vi "main.vi"() -> ()   [LabVIEW 2017]
panel:
  in  "stop get state":bool
  out "Robot mode":T1(ring)
  out "client out byte array":u8[](array[numeric])
  out "state client out":string
  out "state error out 2":errorcluster
  out "Robot mode":T1(ring)
  out "speed cmd string":string
  out "JointMovJ string":string
  in  "j4-":bool
  in  "j3-":bool
  in  "j2-":bool
  in  "j1-":bool
  in  "j4+":bool
  in  "j3+":bool
  in  "j2+":bool
  in  "j1+":bool
  out "client out byte array":u8[](array[numeric])
  out "state error out":errorcluster
  out "state client out":string
  in  "Robot State":bool
  out "error out":errorcluster
  in  "Start trace":bool
  in  "tracePath":string
  in  "Stop move":bool
  in  "JointMovJ":bool
  in  "j4":dbl
  in  "j3":dbl=100.0
  in  "j2":dbl
  in  "j1":dbl
  in  "Speed confrim":bool
  in  "Speed Factor":dbl
  in  "Emergency Stop":bool
  in  "Power up":bool
  out "data out":string
  in  "ClearError":bool
  in  "Enable button":bool
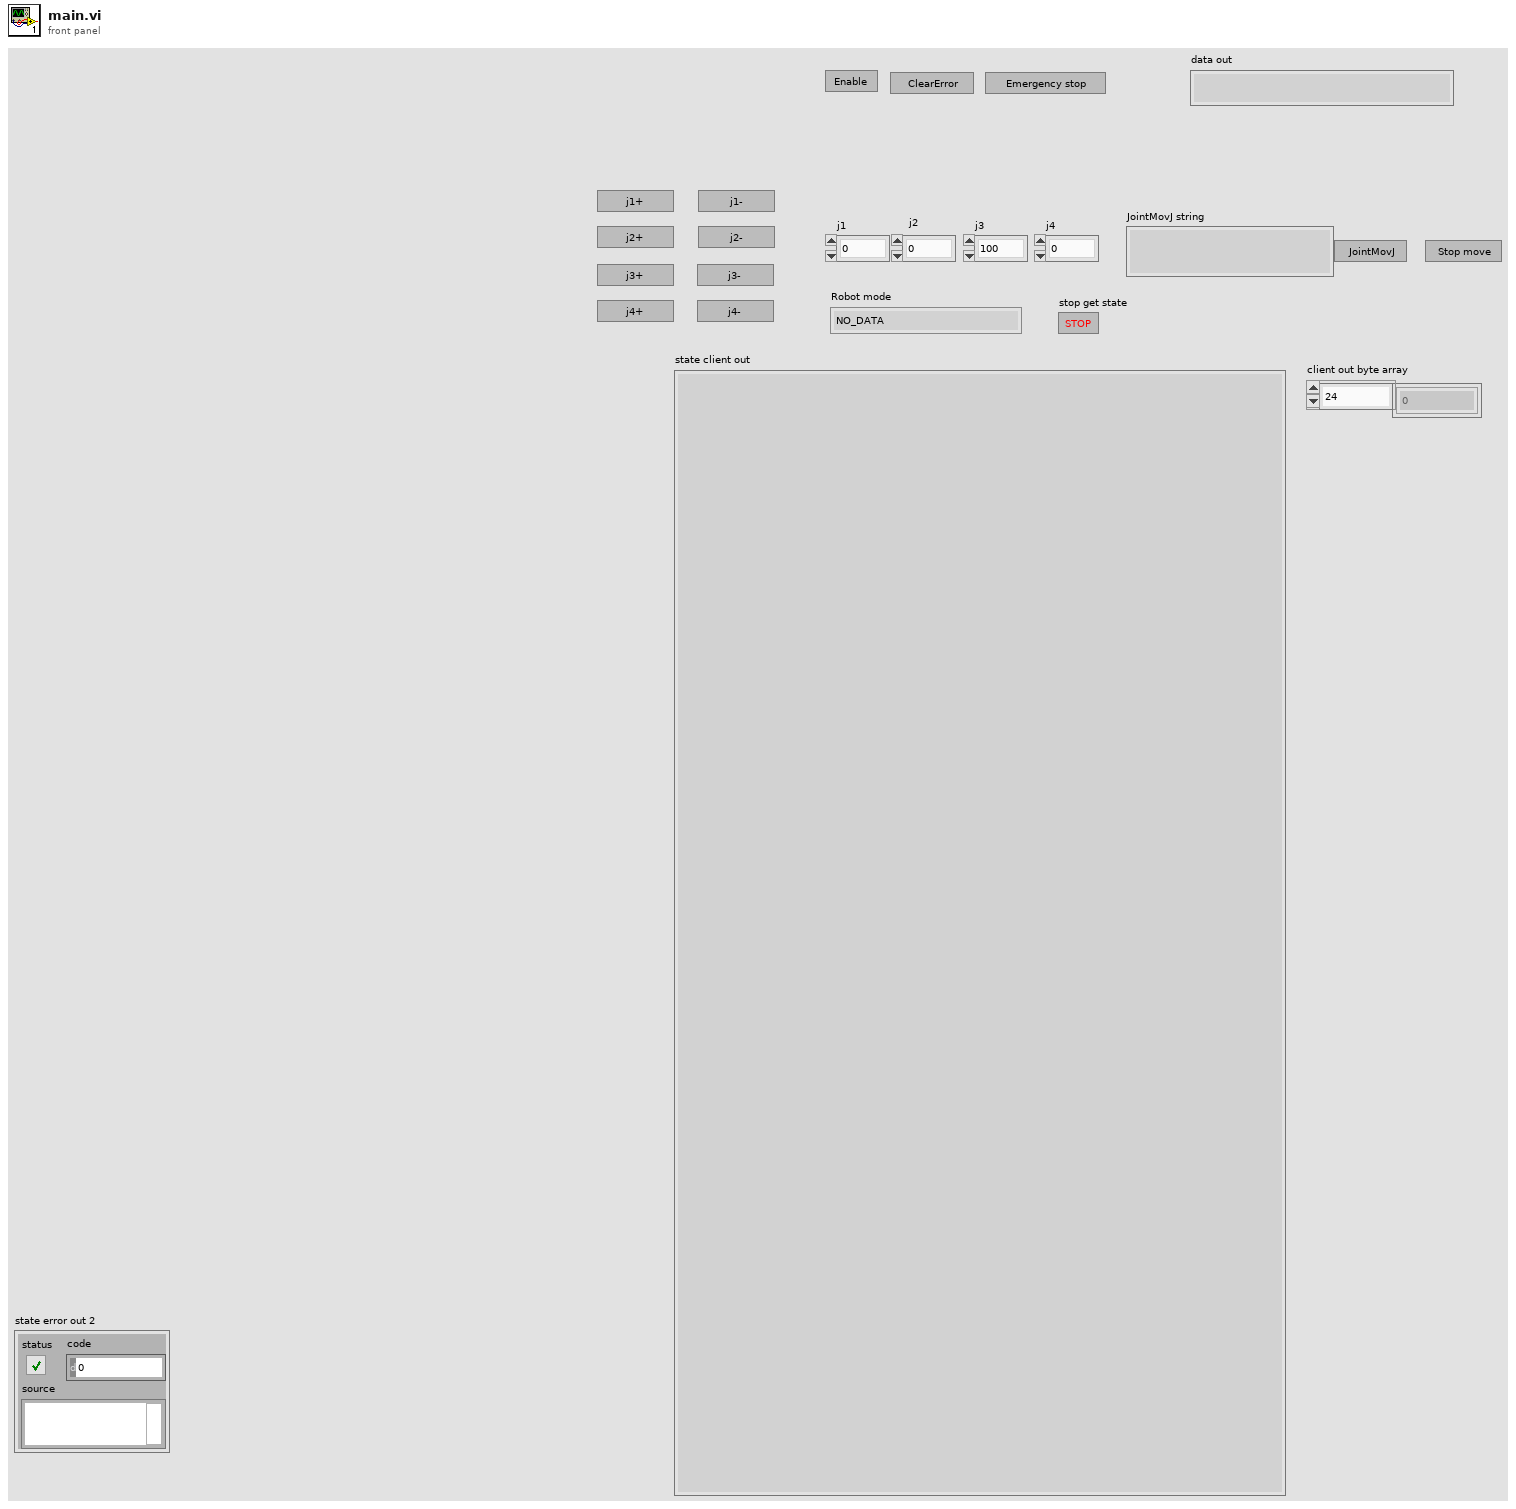
[diagram p1: front panel]
types:
  T1 = enum16{"NO_DATA", "ROBOT_MODE_INIT", "ROBOT_MODE_BRAKE_OPEN", "HOLD_BITS", "ROBOT_MODE_DISABLED", "ROBOT_MODE_ENABLE", "ROBOT_MODE_BACKDRIVE", "ROBOT_MODE_RUNNING", "ROBOT_MODE_RECORDING", "ROBOT_MODE_ERROR", "ROBOT_MODE_PAUSE", "ROBOT_MODE_JOG"}
  T2 = enum16{"Standard", "Buffered", "CRLF", "Immediate"}
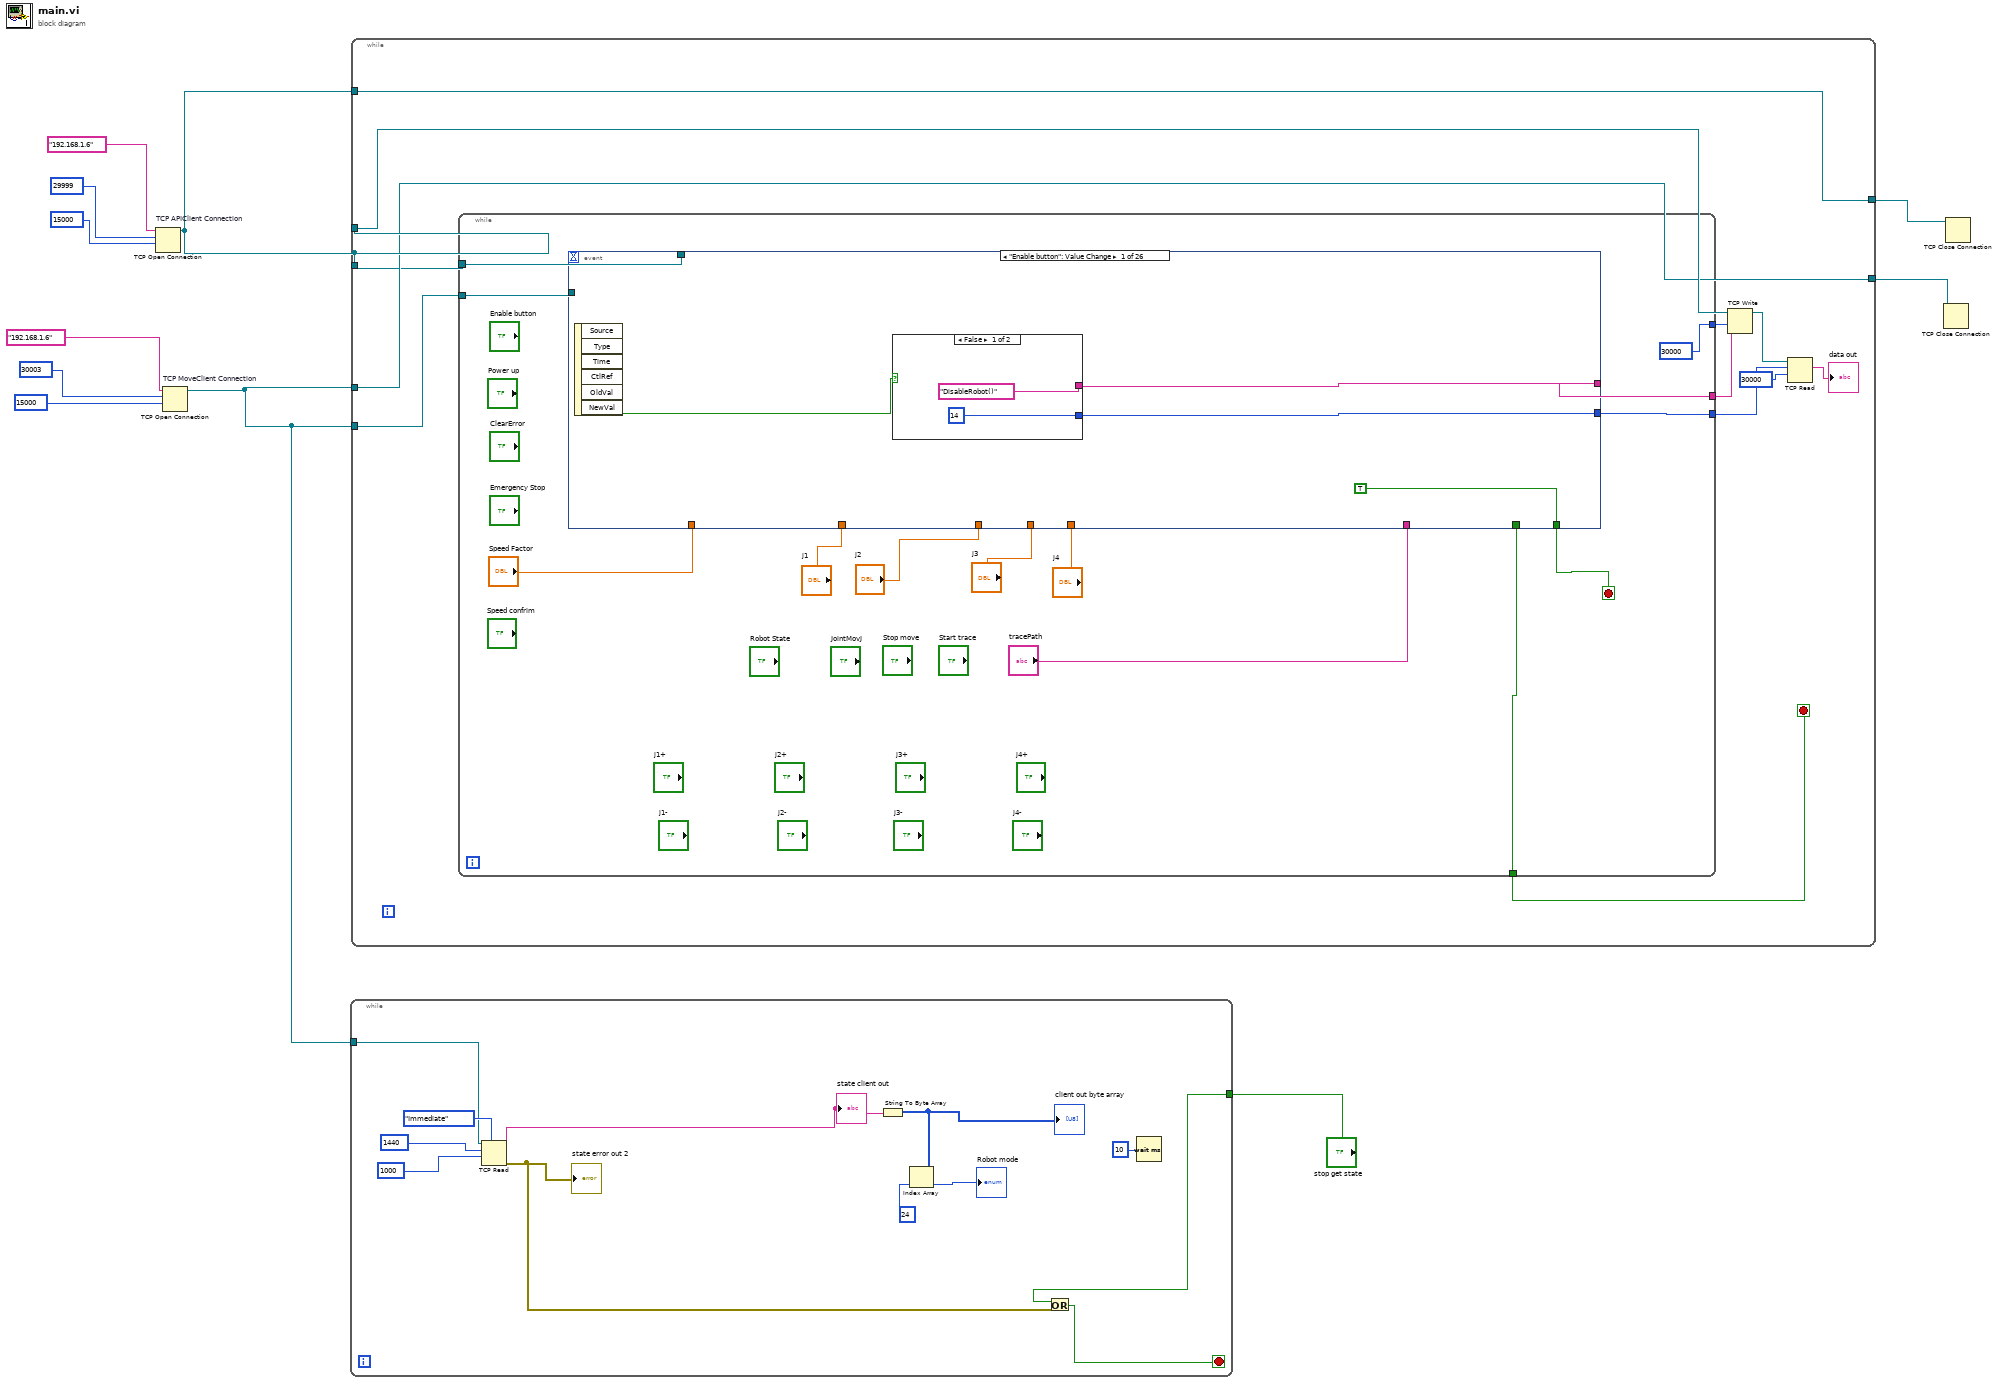
[diagram p0: block diagram]
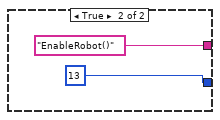
[diagram p2: hidden frame]
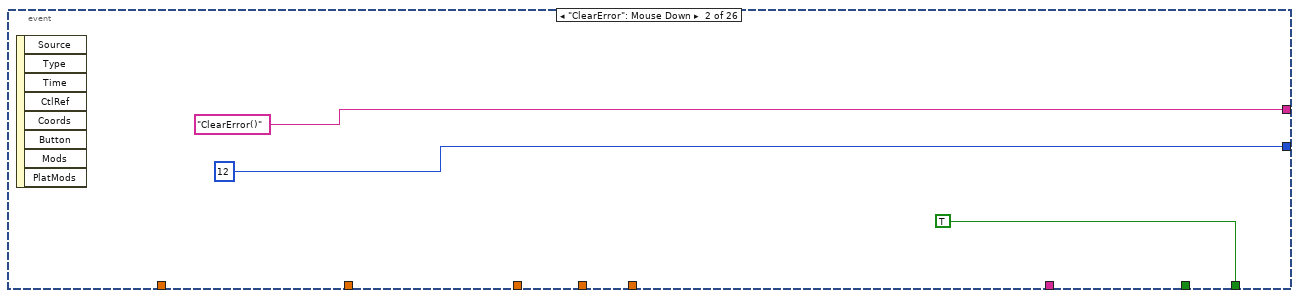
[diagram p3: hidden frame]
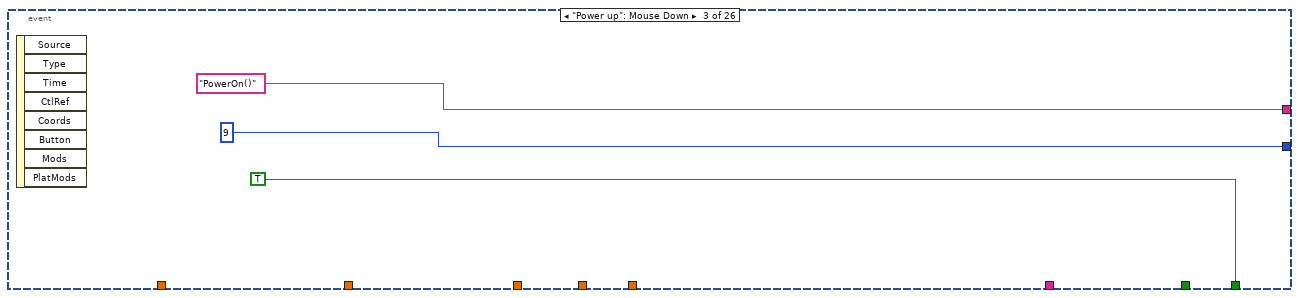
[diagram p4: hidden frame]
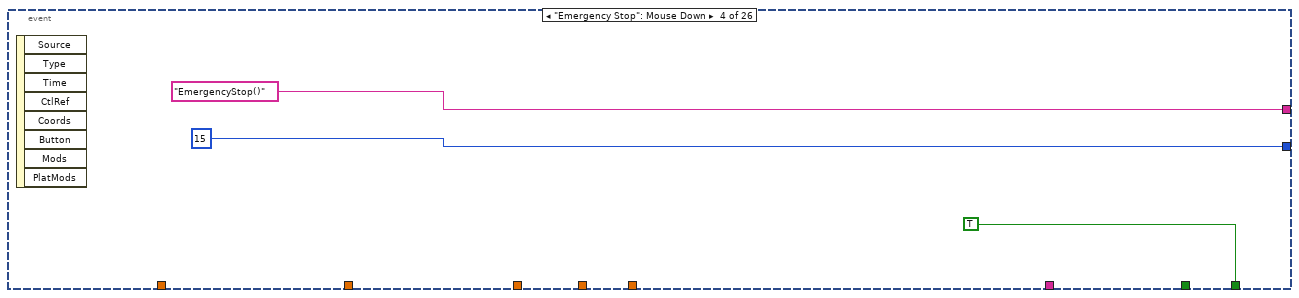
[diagram p5: hidden frame]
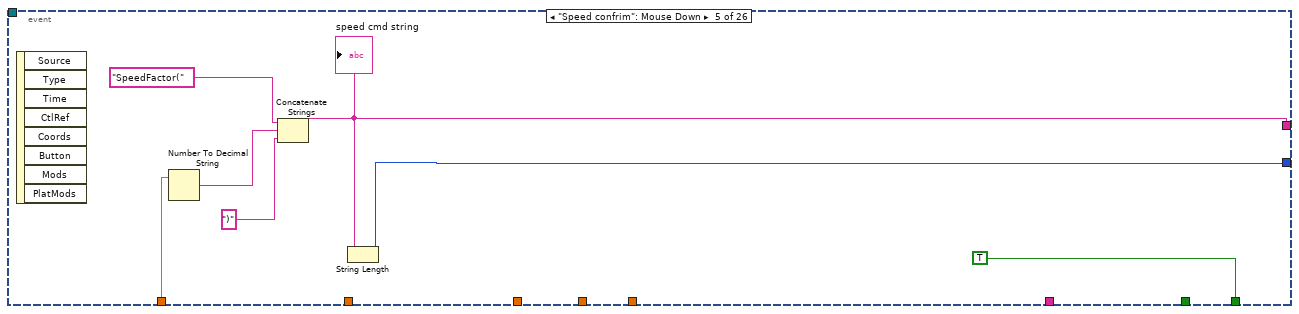
[diagram p6: hidden frame]
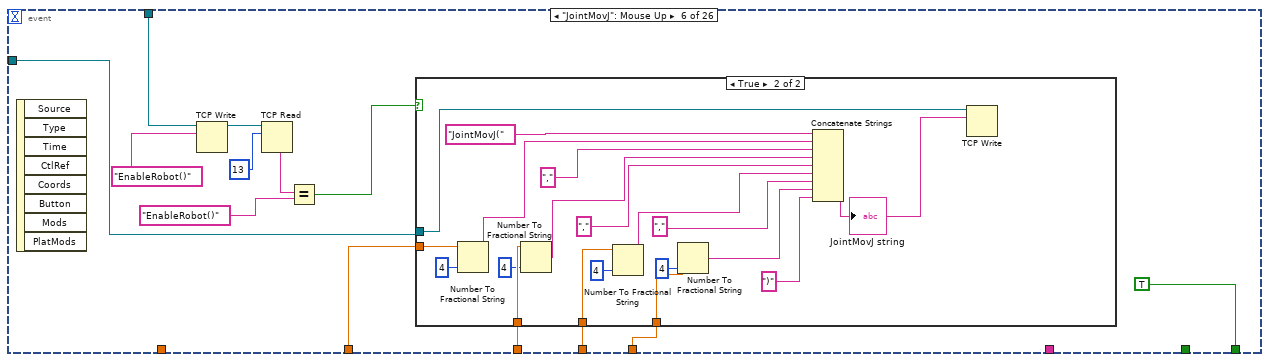
[diagram p7: hidden frame]
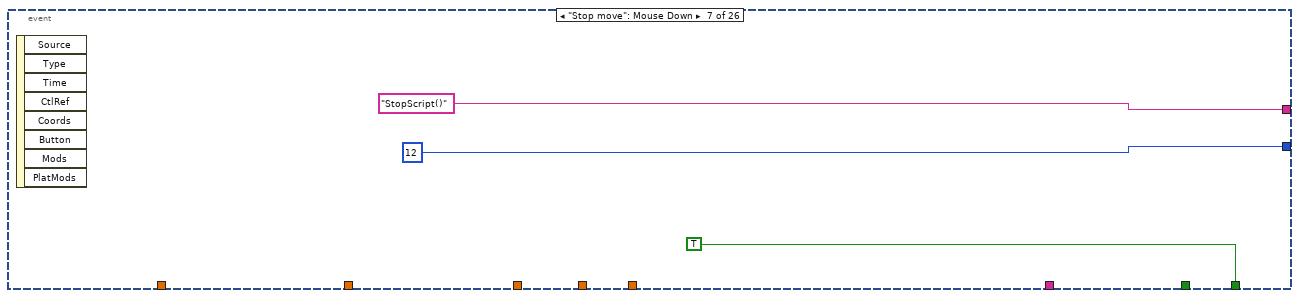
[diagram p9: hidden frame]
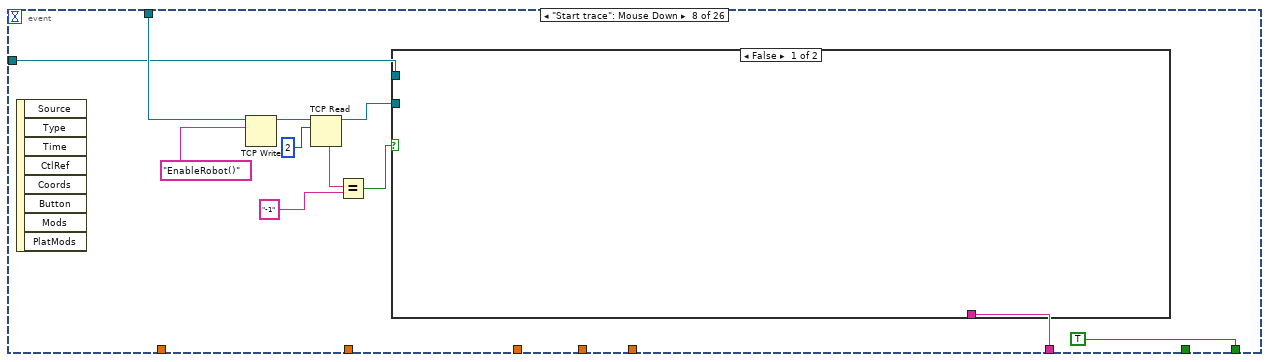
[diagram p10: hidden frame]
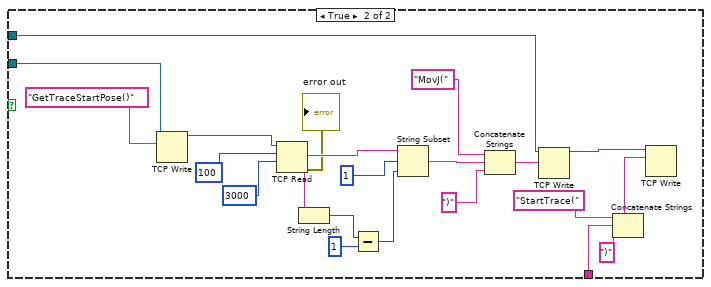
[diagram p11: hidden frame]
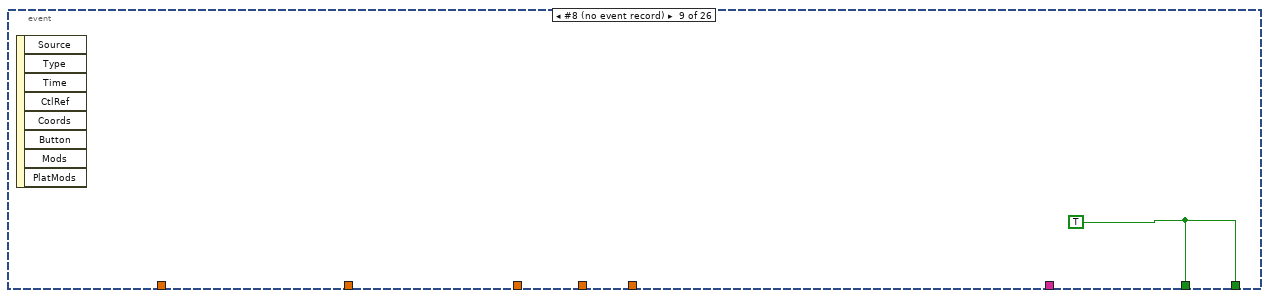
[diagram p12: hidden frame]
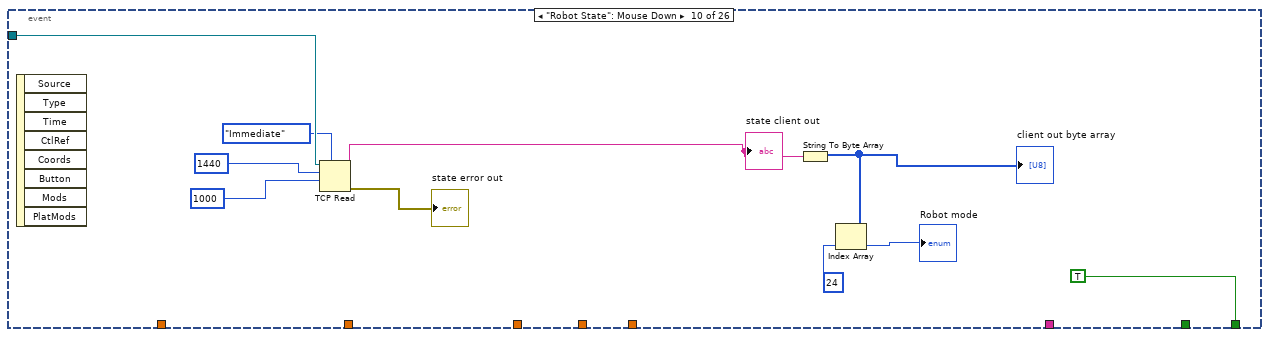
[diagram p13: hidden frame]
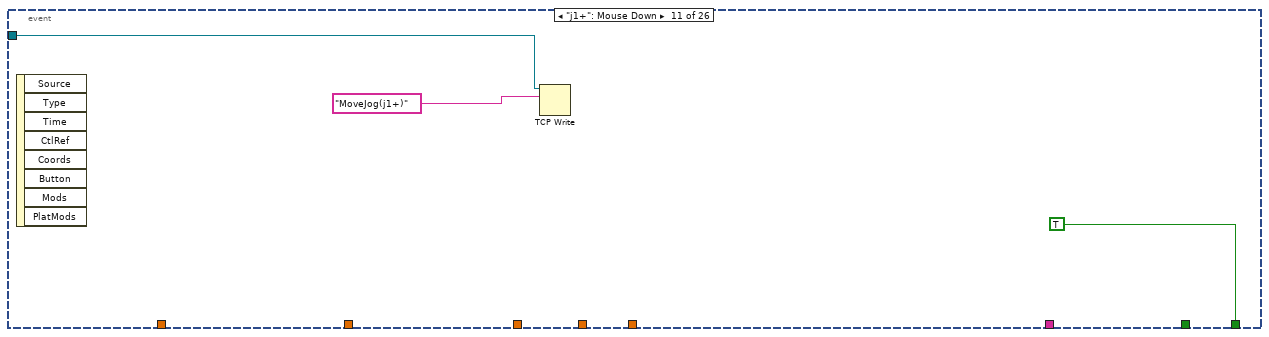
[diagram p14: hidden frame]
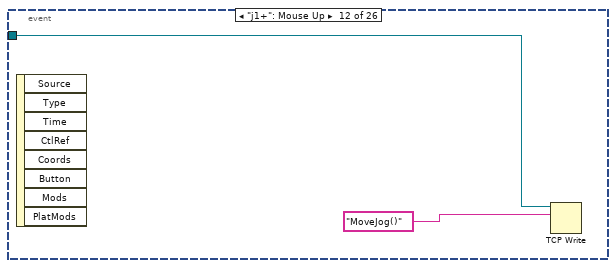
[diagram p15: hidden frame]
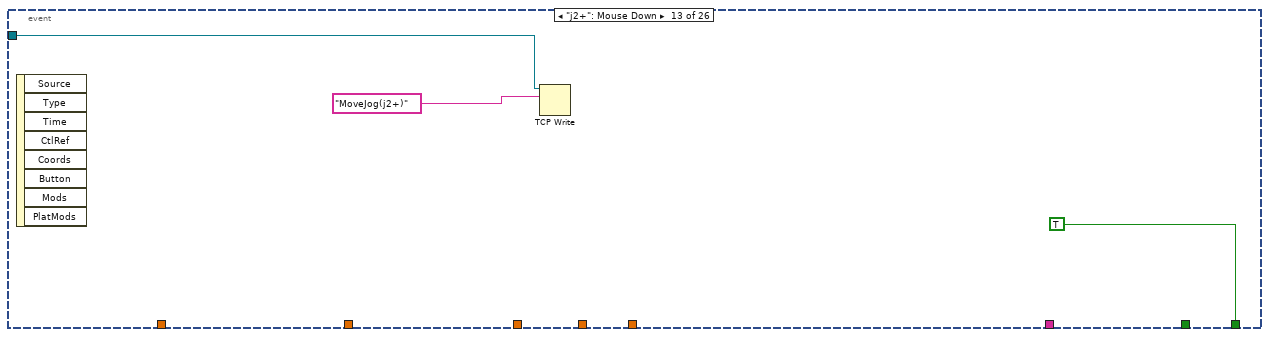
[diagram p16: hidden frame]
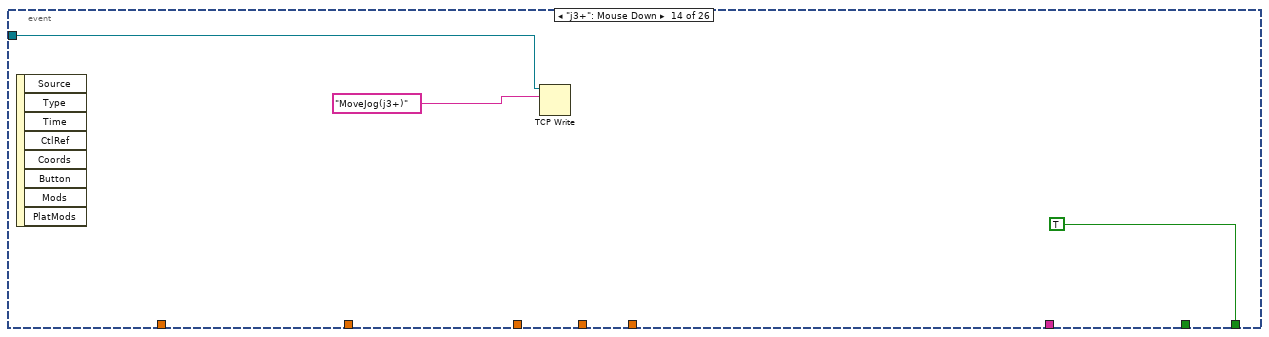
[diagram p17: hidden frame]
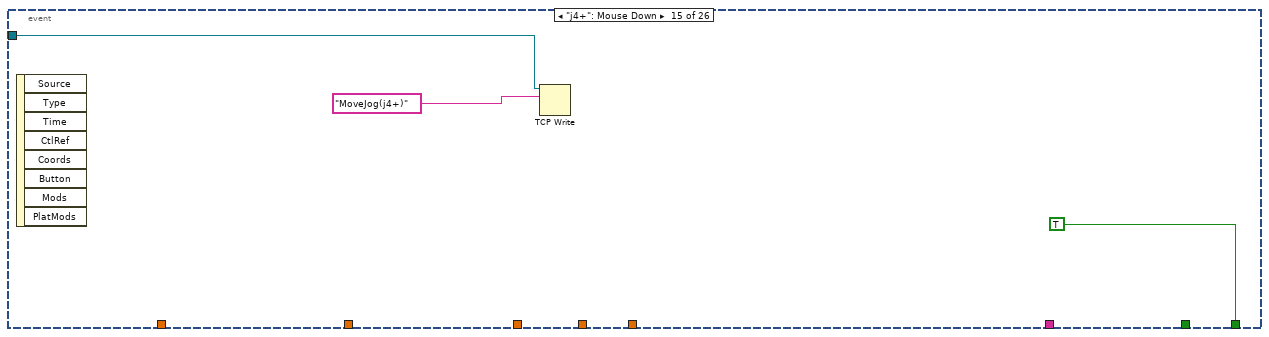
[diagram p18: hidden frame]
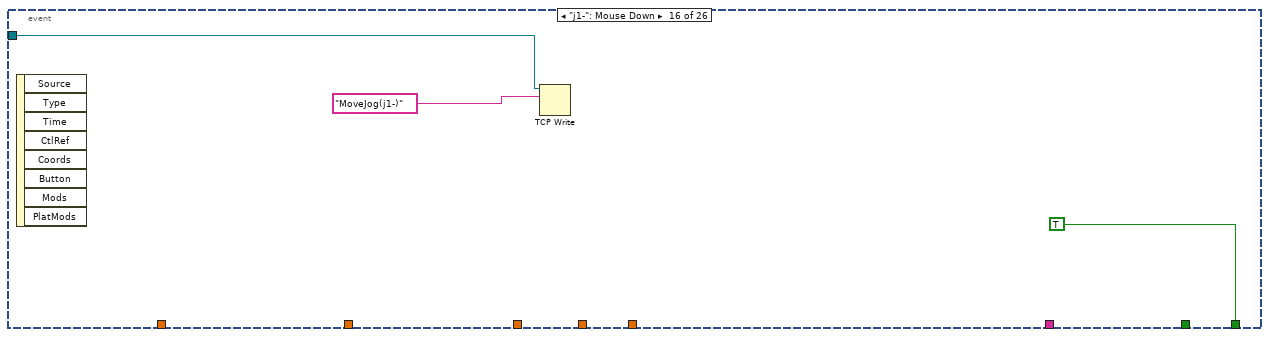
[diagram p19: hidden frame]
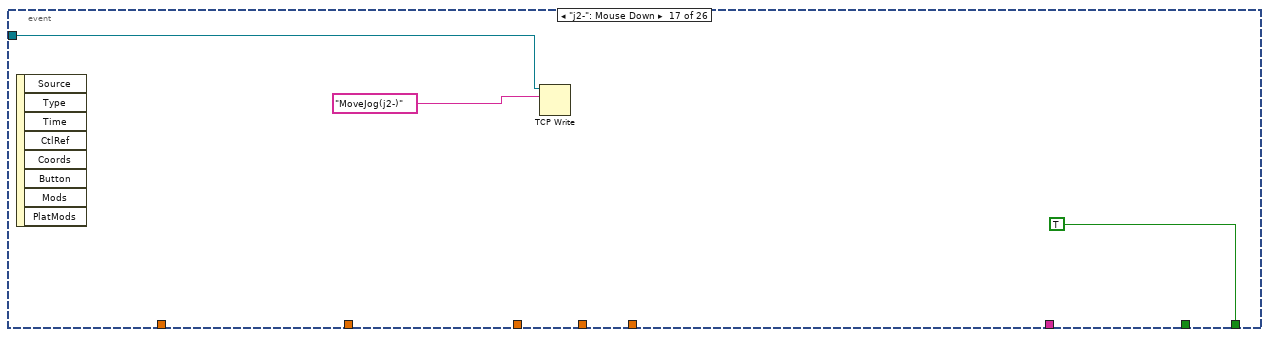
[diagram p20: hidden frame]
diagram:
  n1 = TCP Open Connection "TCP APIClient Connection"(address="192.168.1.6", remote port or service name=29999, timeout ms (60000)=15000) -> (connection ID=w3:refnum<k5>)  [unwired: 2 in, 1 out]
  n2 = TCP Open Connection "TCP MoveClient Connection"(address="192.168.1.6", remote port or service name=30003, timeout ms (60000)=15000) -> (connection ID=w2:refnum<k5>)  [unwired: 2 in, 1 out]
  n3 = while {
    tunnel: w2 -> [w20]
    tunnel: "stop get state" -> [w14]
    stop <- w13 stop-if-true
    n4 = TCP Read(connection ID=w20, bytes to read=1440, 7:T2."Immediate" ("mode (standard)"), 9:1000 ("timeout ms (25000)")) -> (data out=w16:string, error out=w12:errorcluster)  [unwired: 1 in, 1 out]
    "state error out 2" <- w12
    "state client out" <- w16
    n5 = String To Byte Array(string=w16) -> (unsigned byte array=w19:u8[])
    "client out byte array" <- w19
    n6 = Index Array(array=w19, index=24) -> (element=→"Robot mode":u8)
    n7 = Or(x=w14, y=w12) -> (x .or. y?=w13:bool)
    n8 = Wait (ms)(milliseconds to wait=u32 10) -> ()  [unwired: 1 out]
  }
  n9 = while {
    tunnel: w3 -> [w34]
    tunnel: [w30] -> w5
    tunnel: w2 -> [w30]
    tunnel: [w29] -> w4
    tunnel: w3 -> [w29]
    tunnel: w3 -> [w28]
    tunnel: w2 -> [w27]
    stop <- w26 stop-if-true
    n10 = while {
      tunnel: [w41] -> w35
      tunnel: [w48] -> w32
      tunnel: w28 -> [w46]
      tunnel: w27 -> [w45]
      tunnel: [w38] -> w26
      tunnel: [30000 ("timeout ms (25000)")] -> w24
      stop <- w39 stop-if-true
      n11 = event shown="[0] \"Enable button\": Value Change" {
        selector: _ -> [_ _ _ _ _ _ _ _ _ _ _ _ _ _ _ _ _ _ _ _ _ _ _ _ _ _]
        dyn-events: _ -> [_ _ _ _ _ _ _ _ _ _ _ _ _ _ _ _ _ _ _ _ _ _ _ _ _ _]
        timeout: _ -> [_ _ _ _ _ _ _ _ _ _ _ _ _ _ _ _ _ _ _ _ _ _ _ _ _ _]
        tunnel: [w52 "ClearError()" "PowerOn()" "EmergencyStop()" w68 _ "StopScript()" _ _ _ _ _ _ _ _ _ _ _ _ _ _ _ _ _ _ _] -> w41
        tunnel: [w51 12 9 15 w70 _ 12 _ _ _ _ _ _ _ _ _ _ _ _ _ _ _ _ _ _ _] -> w48
        tunnel: "Speed Factor" -> [_ _ _ _ w72 _ _ _ _ _ _ _ _ _ _ _ _ _ _ _ _ _ _ _ _ _]
        tunnel: w46 -> [_ _ _ _ _ w85 _ w113 _ _ _ _ _ _ _ _ _ _ _ _ _ _ _ _ _ _]
        tunnel: w45 -> [_ _ _ _ _ w79 _ w110 _ w146 w151 w154 w156 w159 w162 w165 w168 w171 w174 w177 w179 w181 w183 w185 w187 w189]
        tunnel: "j1" -> [_ _ _ _ _ w78 _ _ _ _ _ _ _ _ _ _ _ _ _ _ _ _ _ _ _ _]
        tunnel: "j2" -> [_ _ _ _ _ w77 _ _ _ _ _ _ _ _ _ _ _ _ _ _ _ _ _ _ _ _]
        tunnel: "j3" -> [_ _ _ _ _ w76 _ _ _ _ _ _ _ _ _ _ _ _ _ _ _ _ _ _ _ _]
        tunnel: "j4" -> [_ _ _ _ _ w75 _ _ _ _ _ _ _ _ _ _ _ _ _ _ _ _ _ _ _ _]
        tunnel: "tracePath" -> [_ _ _ _ _ _ _ w109 _ _ _ _ _ _ _ _ _ _ _ _ _ _ _ _ _ _]
        tunnel: [TRUE TRUE TRUE TRUE TRUE TRUE TRUE TRUE w140 TRUE TRUE _ TRUE TRUE TRUE TRUE TRUE TRUE TRUE _ _ _ _ _ _ _] -> w39
        tunnel: [_ _ _ _ _ _ _ _ w140 _ _ _ _ _ _ _ _ _ _ _ _ _ _ _ _ _] -> w38
        event "Enable button": Value Change {
          n12 = event-data() -> ("NewVal"=w49:bool)  [unwired: 1 in, 5 out]
          n13 = case shown="False" w49 {
            tunnel: ["DisableRobot()" "EnableRobot()"] -> w52
            tunnel: [14 13] -> w51
            frame False {
            }
            frame True {
            }
          }
        }
        event "ClearError": Mouse Down {
          n14 = event-data() -> ()  [unwired: 1 in, 8 out]
        }
        event "Power up": Mouse Down {
          n15 = event-data() -> ()  [unwired: 1 in, 8 out]
        }
        event "Emergency Stop": Mouse Down {
          n16 = event-data() -> ()  [unwired: 1 in, 8 out]
        }
        event "Speed confrim": Mouse Down {
          n17 = event-data() -> ()  [unwired: 1 in, 8 out]
          n18 = Number To Decimal String(number=w72) -> (decimal integer string=w67:string)  [unwired: 1 in]
          n19 = Concatenate Strings("SpeedFactor(", w67, ")") -> (w68:string)
          "speed cmd string" <- w68
          n20 = String Length(string=w68) -> (length=w70:i32)
        }
        event "JointMovJ": Mouse Up {
          n21 = event-data() -> ()  [unwired: 1 in, 8 out]
          n22 = TCP Write(connection ID=w85, data in="EnableRobot()") -> (connection ID out=w84:refnum<k5>)  [unwired: 2 in, 2 out]
          n23 = TCP Read(connection ID=w84, bytes to read=13) -> (data out=w81:string)  [unwired: 3 in, 2 out]
          n24 = Equal?(x=w81, y="EnableRobot()") -> (x = y?=w74:bool)
          n25 = case shown="True" w74 {
            tunnel: w79 -> [_ w104]
            tunnel: w78 -> [_ w103]
            tunnel: w77 -> [_ w102]
            tunnel: w76 -> [_ w101]
            tunnel: w75 -> [_ w100]
            frame False {
            }
            frame True {
              n26 = Number To Fractional String(number=w103, precision (6)=i16 4) -> (F-format string=w99:string)  [unwired: 2 in]
              n27 = Number To Fractional String(number=w102, precision (6)=i16 4) -> (F-format string=w95:string)  [unwired: 2 in]
              n28 = Number To Fractional String(number=w101, precision (6)=i16 4) -> (F-format string=w91:string)  [unwired: 2 in]
              n29 = Number To Fractional String(number=w100, precision (6)=i16 4) -> (F-format string=w93:string)  [unwired: 2 in]
              n30 = Concatenate Strings("JointMovJ(" ("string"), w99, "," ("string"), w95, "," ("string"), w91, "," ("string"), w93, ")" ("string")) -> (w86:string)
              "JointMovJ string" <- w86
              n31 = TCP Write(connection ID=w104, data in=w86) -> ()  [unwired: 2 in, 3 out]
            }
          }
        }
        event "Stop move": Mouse Down {
          n32 = event-data() -> ()  [unwired: 1 in, 8 out]
        }
        event "Start trace": Mouse Down {
          n33 = event-data() -> ()  [unwired: 1 in, 8 out]
          n34 = TCP Write(connection ID=w113, data in="EnableRobot()") -> (connection ID out=w118:refnum<k5>)  [unwired: 2 in, 2 out]
          n35 = TCP Read(connection ID=w118, bytes to read=2) -> (connection ID out=w111:refnum<k5>, data out=w115:string)  [unwired: 3 in, 1 out]
          n36 = Equal?(x=w115, y="-1") -> (x = y?=w112:bool)
          n37 = case shown="False" w112 {
            tunnel: w111 -> [_ w138]
            tunnel: w110 -> [_ w125]
            tunnel: w109 -> [_ w121]
            frame False {
            }
            frame True {
              n38 = TCP Write(connection ID=w138, data in="GetTraceStartPose()") -> (connection ID out=w136:refnum<k5>)  [unwired: 2 in, 2 out]
              n39 = TCP Read(connection ID=w136, bytes to read=100, 9:3000 ("timeout ms (25000)")) -> (data out=w133:string, error out=→"error out":errorcluster)  [unwired: 2 in, 1 out]
              n40 = String Length(string=w133) -> (length=w132:i32)
              n41 = Subtract(x=w132, y=1) -> (x-y=w130:i32)
              n42 = String Subset(string=w133, offset (0)=1, length (rest)=w130) -> (substring=w128:string)
              n43 = Concatenate Strings("MovJ(" ("string"), w128, ")" ("string")) -> (w126:string)
              n44 = TCP Write(connection ID=w125, data in=w126) -> (connection ID out=w124:refnum<k5>)  [unwired: 2 in, 2 out]
              n45 = Concatenate Strings("StartTrace(" ("string"), w121, ")" ("string")) -> (w122:string)
              n46 = TCP Write(connection ID=w124, data in=w122) -> ()  [unwired: 2 in, 3 out]
            }
          }
        }
        event #8 (no event record) {
          w140 = TRUE
          n47 = event-data() -> ()  [unwired: 1 in, 8 out]
        }
        event "Robot State": Mouse Down {
          n48 = event-data() -> ()  [unwired: 1 in, 8 out]
          n49 = TCP Read(connection ID=w146, bytes to read=1440, 7:T2."Immediate" ("mode (standard)"), 9:1000 ("timeout ms (25000)")) -> (data out=w145:string, error out=→"state error out":errorcluster)  [unwired: 1 in, 1 out]
          "state client out" <- w145
          n50 = String To Byte Array(string=w145) -> (unsigned byte array=w144:u8[])
          "client out byte array" <- w144
          n51 = Index Array(array=w144, index=24) -> (element=→"Robot mode":u8)
        }
        event "j1+": Mouse Down {
          n52 = event-data() -> ()  [unwired: 1 in, 8 out]
          n53 = TCP Write(connection ID=w151, data in="MoveJog(j1+)") -> ()  [unwired: 2 in, 3 out]
        }
        event "j1+": Mouse Up {
          n54 = event-data() -> ()  [unwired: 1 in, 8 out]
          n55 = TCP Write(connection ID=w154, data in="MoveJog()") -> ()  [unwired: 2 in, 3 out]
        }
        event "j2+": Mouse Down {
          n56 = event-data() -> ()  [unwired: 1 in, 8 out]
          n57 = TCP Write(connection ID=w156, data in="MoveJog(j2+)") -> ()  [unwired: 2 in, 3 out]
        }
        event "j3+": Mouse Down {
          n58 = event-data() -> ()  [unwired: 1 in, 8 out]
          n59 = TCP Write(connection ID=w159, data in="MoveJog(j3+)") -> ()  [unwired: 2 in, 3 out]
        }
        event "j4+": Mouse Down {
          n60 = event-data() -> ()  [unwired: 1 in, 8 out]
          n61 = TCP Write(connection ID=w162, data in="MoveJog(j4+)") -> ()  [unwired: 2 in, 3 out]
        }
        event "j1-": Mouse Down {
          n62 = event-data() -> ()  [unwired: 1 in, 8 out]
          n63 = TCP Write(connection ID=w165, data in="MoveJog(j1-)") -> ()  [unwired: 2 in, 3 out]
        }
        event "j2-": Mouse Down {
          n64 = event-data() -> ()  [unwired: 1 in, 8 out]
          n65 = TCP Write(connection ID=w168, data in="MoveJog(j2-)") -> ()  [unwired: 2 in, 3 out]
        }
        event "j3-": Mouse Down {
          n66 = event-data() -> ()  [unwired: 1 in, 8 out]
          n67 = TCP Write(connection ID=w171, data in="MoveJog(j3-)") -> ()  [unwired: 2 in, 3 out]
        }
        event "j4-": Mouse Down {
          n68 = event-data() -> ()  [unwired: 1 in, 8 out]
          n69 = TCP Write(connection ID=w174, data in="MoveJog(j4-)") -> ()  [unwired: 2 in, 3 out]
        }
        event "j2+": Mouse Up {
          n70 = event-data() -> ()  [unwired: 1 in, 8 out]
          n71 = TCP Write(connection ID=w177, data in="MoveJog()") -> ()  [unwired: 2 in, 3 out]
        }
        event "j3+": Mouse Up {
          n72 = event-data() -> ()  [unwired: 1 in, 8 out]
          n73 = TCP Write(connection ID=w179, data in="MoveJog()") -> ()  [unwired: 2 in, 3 out]
        }
        event "j4+": Mouse Up {
          n74 = event-data() -> ()  [unwired: 1 in, 8 out]
          n75 = TCP Write(connection ID=w181, data in="MoveJog()") -> ()  [unwired: 2 in, 3 out]
        }
        event "j1-": Mouse Up {
          n76 = event-data() -> ()  [unwired: 1 in, 8 out]
          n77 = TCP Write(connection ID=w183, data in="MoveJog()") -> ()  [unwired: 2 in, 3 out]
        }
        event "j2-": Mouse Up {
          n78 = event-data() -> ()  [unwired: 1 in, 8 out]
          n79 = TCP Write(connection ID=w185, data in="MoveJog()") -> ()  [unwired: 2 in, 3 out]
        }
        event "j3-": Mouse Up {
          n80 = event-data() -> ()  [unwired: 1 in, 8 out]
          n81 = TCP Write(connection ID=w187, data in="MoveJog()") -> ()  [unwired: 2 in, 3 out]
        }
        event "j4-": Mouse Up {
          n82 = event-data() -> ()  [unwired: 1 in, 8 out]
          n83 = TCP Write(connection ID=w189, data in="MoveJog()") -> ()  [unwired: 2 in, 3 out]
        }
      }
    }
    n84 = TCP Write(connection ID=w34, data in=w35, 9:w24) -> (connection ID out=w33:refnum<k5>)  [unwired: 1 in, 2 out]
    n85 = TCP Read(connection ID=w33, bytes to read=w32, 9:30000 ("timeout ms (25000)")) -> (data out=→"data out":string)  [unwired: 2 in, 2 out]
  }
  n86 = TCP Close Connection(connection ID=w5) -> ()  [unwired: 2 in, 2 out]
  n87 = TCP Close Connection(connection ID=w4) -> ()  [unwired: 2 in, 2 out]
